vi "Dead Reckoning.vi"(8 "Path":dbl[](array[numeric]), 9 "Yaw angle":dbl, 10 "use PID":bool, 11 "Velocity":dbl) -> (0 "Yaw with offset":dbl, 1 "Reference yaw":dbl, 2 "Run dead reckoning?":bool, 3 "Reference lean":dbl, 4 "case":dbl)   [LabVIEW 2016]
uses:
  <vilib>/Simulation/Shared/_Datatypes/SIM SISO Transfer Function.ctl
  <vilib>/Simulation/DiscreteLinear/Implementation/NILVSim Discrete Transfer Function Direct.llb/SIM Discrete Transfer Function Diagram (SISO).vi
  <vilib>/Simulation/ContinuousLinear/Implementation/Shared/SIM Transfer Function Support.llb/SIM TransferFunction Normalize to Buffer.vi
  <vilib>/Simulation/DiscreteLinear/Implementation/Shared/SIM Init Discrete States.vi
  <vilib>/Simulation/DiscreteLinear/Implementation/NILVSim Discrete Transfer Function Direct.llb/SIM Transfer Function Direct core (SISO).vi
  <vilib>/Simulation/ContinuousLinear/Implementation/Shared/SIM Transfer Function Support.llb/SIM TransferFunction Normalize.vi
  <vilib>/Simulation/Implementation/Shared/SIM Polynomials.llb/SIM Remove Zero Coefficients (DBL).vi
  <vilib>/Simulation/Implementation/Shared/SIM Polynomials.llb/SIM Divide Polynomials (DBL).vi
  <vilib>/Simulation/Implementation/Shared/SIM BuildSimErr.vi
  <vilib>/Simulation/Implementation/XNodeFramework/SimXNode/SimX.xnode
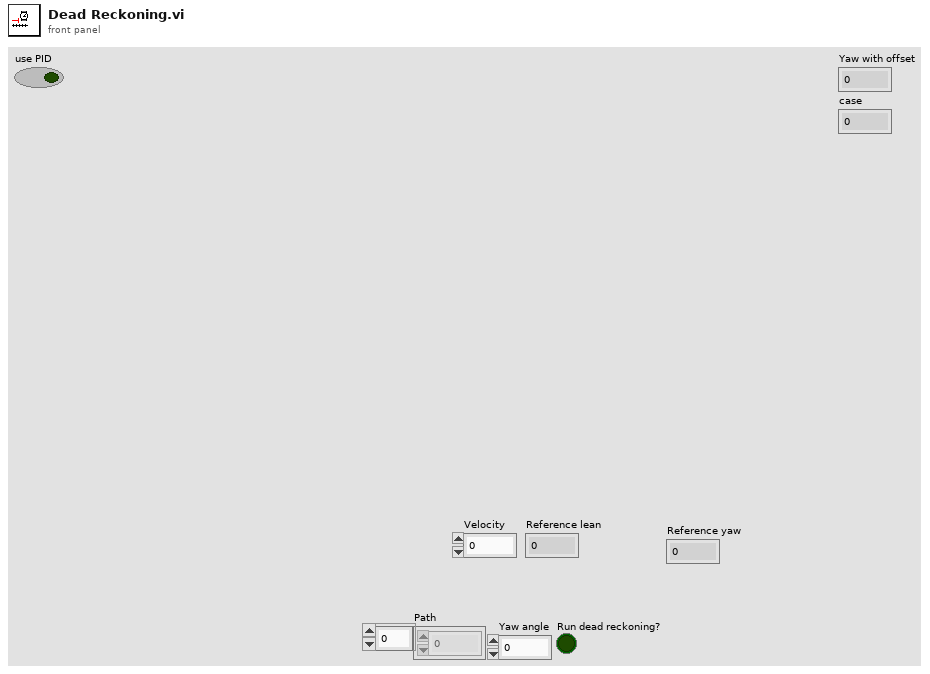
[diagram p1: front panel]
types:
  T1 = cluster{"proportional gain (Kc)":dbl, "integral time (Ti, min)":dbl, "derivative time (Td, min)":dbl}
  T2 = typedef "SIM SISO Transfer Function.ctl" = cluster{"Numerator":dbl[], "Denominator":dbl[]}
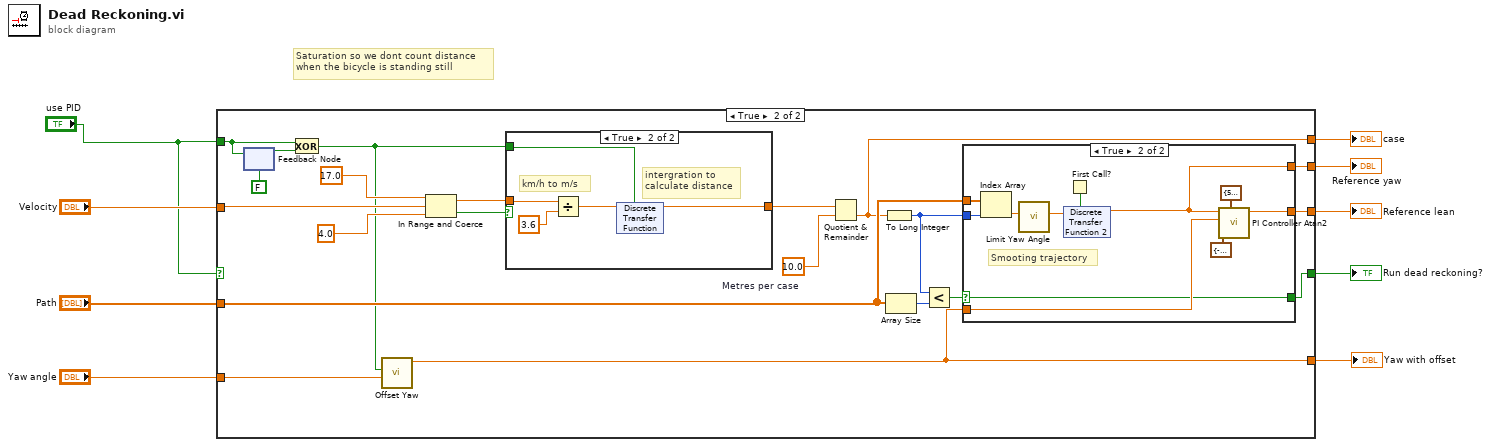
[diagram p0: block diagram]
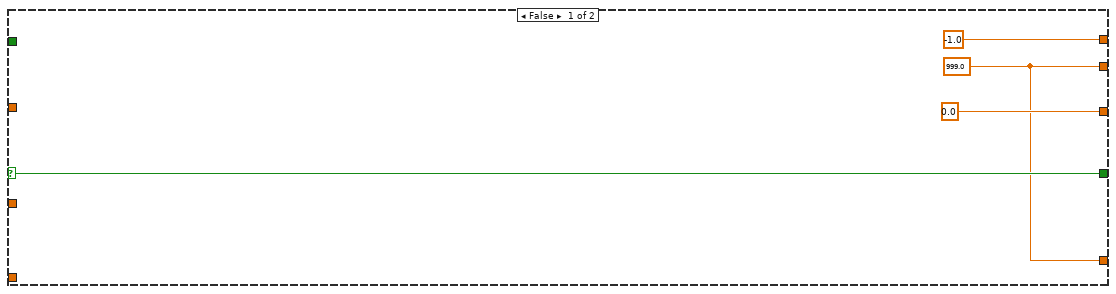
[diagram p2: hidden frame]
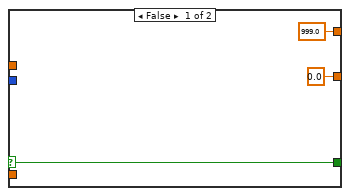
[diagram p3: hidden frame]
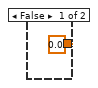
[diagram p4: hidden frame]
diagram:
  # "Saturation so we dont count distance\nwhen the bicycle is standing still"
  n1 = case shown="True" "use PID" {
    selector: "use PID" -> [w11 _]
    tunnel: "use PID" -> [_ w23]
    tunnel: "Velocity" -> [_ w26]
    tunnel: "Path" -> [_ w25]
    tunnel: "Yaw angle" -> [_ w19]
    tunnel: [0.0 ("output") w24] -> w6
    tunnel: [w10 w18] -> w5
    tunnel: [-1.0 w14] -> w4
    tunnel: [w10 w16] -> w3
    tunnel: [w11 w15] -> w2
    frame False {
      w10 = 999.0 ("output y(k)")
    }
    frame True {
      w17 = 10.0  # Metres per case
      n2 = feedback #1(FALSE) -> (w30:bool)
      n3 = feedback-in #1(w23) -> ()
      n4 = Exclusive Or(1:w30, 2:w23) -> (0:w20:bool)
      n5 = call "Offset Yaw.vi"("Sensor Yaw"=w19, "Trigger offset"=w20) -> ("Yaw with offset"=w18:dbl)  [unwired: 9 in]
      n6 = In Range and Coerce(upper limit=17.0, x=w26, lower limit=4.0) -> (coerced(x)=w31:dbl, In Range?=w32:bool)
      n7 = case shown="True" w32 {
        tunnel: w31 -> [_ w59]
        tunnel: w20 -> [_ w57]
        tunnel: [0.0 w56] -> w28
        frame False {
        }
        frame True {
          # "intergration to \ncalculate distance"
          # "km/h to m/s"
          n8 = Divide(x=w59, y=3.6) -> (x/y=w58:dbl)
          n9 = xnode "Discrete Transfer Function"("input u(k)"=w58, "initialize"=w57) -> ("output y(k)"=w56:dbl)  [unwired: 1 in, 1 out]
        }
      }
      n10 = Quotient & Remainder(x=w28, y=w17) -> (floor(x/y)=w14:dbl)  [unwired: 1 out]
      n11 = To Long Integer(number=w14) -> (32bit integer=w21:i32)
      n12 = Array Size(array=w25) -> (size(s)=w27:i32)
      n13 = Less?(x=w21, y=w27) -> (x < y?=w22:bool)
      n14 = case shown="True" w22 {
        selector: w22 -> [w35 w38]
        tunnel: w21 -> [_ w48]
        tunnel: w25 -> [_ w47]
        tunnel: w18 -> [_ w43]
        tunnel: [0.0 ("output") w40] -> w24
        tunnel: [999.0 ("output y(k)") w39] -> w16
        tunnel: [w35 w38] -> w15
        frame False {
        }
        frame True {
          # "Smooting trajectory"
          n15 = Index Array(array=w47, index=w48) -> (element=w46:dbl)
          n16 = call "Limit Yaw Angle.vi"("u"=w46) -> ("output"=w45:dbl)  [unwired: 10 in]
          n17 = First Call?() -> (First Call?: T/F=w44:bool)
          n18 = xnode ("Discrete Transfer Function 2")("input u(k)"=w45, "initialize"=w44) -> ("output y(k)"=w39:dbl)  [unwired: 1 in, 1 out]
          n19 = call "PI Controller Atan2.vi"("output range"=cluster{"output high":dbl, "output low":dbl} {"output high"=5.0, "output low"=-5.0}, "PID gains"=T1 {"proportional gain (Kc)"=-0.07592, "integral time (Ti, min)"=157.202, "derivative time (Td, min)"=0.0}, "process variable"=w43, "setpoint"=w39) -> ("output"=w40:dbl)  [unwired: 6 in, 1 out]
        }
      }
    }
  }
  "Reference lean" <- w6
  "Run dead reckoning?" <- w2
  "Reference yaw" <- w3
  "Yaw with offset" <- w5
  "case" <- w4
